vi "Request Node Info.vi"(8 "error in (no error)":errorcluster, 9 "Timeout mS (1000)":i32=1000, 11 "InfoService in":refnum<class "NodeStatus.lvclass">) -> (0 "error out":errorcluster, 2 "Node Info":T1, 3 "InfoService out":refnum<class "NodeStatus.lvclass">)   [LabVIEW 2020, in "Vecto.lvlib" / "NodeStatus.lvclass"]
uses:
  NodeStatus.lvclass
  Node Info.ctl
  Task Info.ctl
  NodeInfoValue/NodeInfoValue.lvclass
  C:/dev/lv20CE/relink/lv-promises/Promises/Value/Value.lvclass
  NodeStatus.lvclass/NodeStatus.ctl
  lv-promises/Promises/Promise/Promise.lvclass/Promise.ctl
  lv-promises/Promises/Future/Future.lvclass/Future.ctl
  NodeInfoValue/NodeInfoValue.lvclass/NodeInfoValue.ctl
  lv-promises/Promises/Future/Future.lvclass
  lv-promises/Promises/Promise/Promise.lvclass
  VectoConfig/VectoConfig.lvlib
  Vecto.lvlib
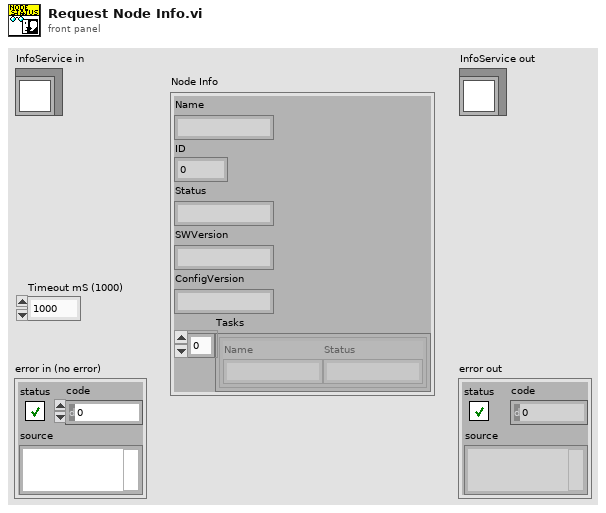
[diagram p1: front panel]
types:
  T1 = typedef "Vecto.lvlib/Node Info.ctl" = cluster{"Name":string, "ID":u32, "Status":string, "SWVersion":string, "ConfigVersion":string, "Tasks":T2[]}
  T2 = typedef "VectoConfig.lvlib/Task Info.ctl" = cluster{"Name":string, "Status":string}
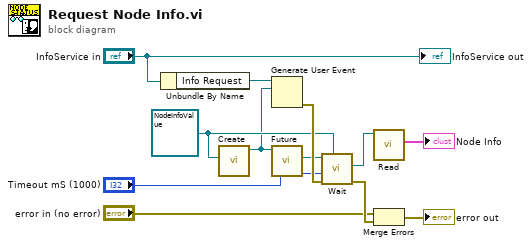
[diagram p0: block diagram]
diagram:
  w9 = refnum<class "NodeInfoValue.lvclass"> refnum ("Vecto.lvlib:NodeInfoValue.lvclass")
  n1 = Unbundle By Name("InfoService in") -> ("Info Request"=w2:refnum<user-event>)
  n2 = call "Create.vi"("Result Type"=w9) -> ("Promise"=w1:refnum<class "Promise.lvclass">)  [unwired: 9 in, 1 out]
  n3 = Generate User Event(user event=w2, event data cluster=w1) -> (error out=w12:errorcluster)  [unwired: 2 in, 1 out]
  n4 = call "Future.vi"("Promise in"=w1) -> ("Future"=w11:refnum<class "Future.lvclass">)  [unwired: 9 in, 1 out]
  n5 = call "Wait.vi"("Result Type"=w9, "error in (no error)"=w12, "Timeout mS (-1)"="Timeout mS (1000)", "Future in"=w11) -> ("error out"=w6:errorcluster, "Result"=w8:refnum<class "NodeInfoValue.lvclass">)  [unwired: 6 in]
  n6 = call "Read.vi"("NodeInfoValue in"=w8) -> ("Node Info"=→"Node Info":T1)  [unwired: 10 in]
  n7 = Merge Errors("error in (no error)", w6) -> (→"error out":errorcluster)
  "InfoService out" <- "InfoService in"
